vi "Structures.vi"() -> ()   [LabVIEW 2020]
panel:
  out "Boolean 4":bool
  out "Boolean 2":bool
  out "for iteration  4":i32
  out "for iteration  2":i32
  in  "Numeric":dbl
  out "for iteration":i32
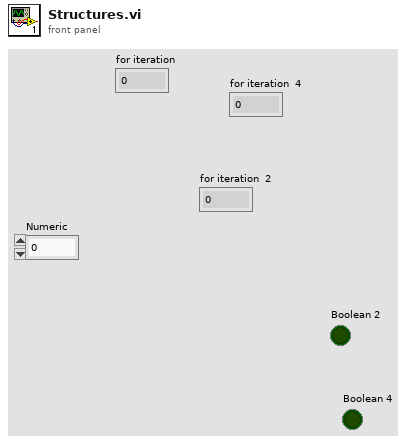
[diagram p1: front panel]
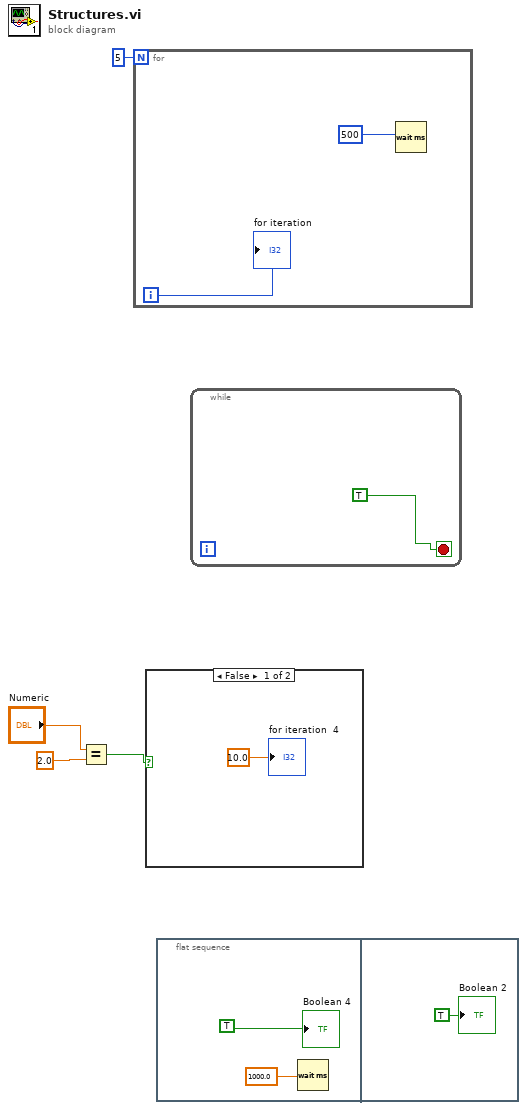
[diagram p0: block diagram]
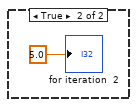
[diagram p2: hidden frame]
diagram:
  n1 = Equal?(x="Numeric", y=2.0) -> (x = y?=w1:bool)
  n2 = for {
    N: 5 -> [_]
    i -> [w6]
    n3 = Wait (ms)(milliseconds to wait=u32 500 ("millisecond timer value")) -> ()  [unwired: 1 out]
    "for iteration" <- w6
  }
  n4 = case shown="False" w1 {
    frame False {
      "for iteration  4" <- 10.0 ("y")
    }
    frame True {
      "for iteration  2" <- 5.0 ("y")
    }
  }
  n5 = flat-sequence {
    frame #0 {
      n6 = Wait (ms)(milliseconds to wait=1000.0 ("y")) -> ()  [unwired: 1 out]
      "Boolean 4" <- TRUE
    }
    frame #1 {
      "Boolean 2" <- TRUE ("Boolean 2")
    }
  }
  n7 = while {
    stop <- TRUE stop-if-true
  }
